vi "VelocityControl.vi"(0 "estimatives":T3, 1 "Dest_orientation":dbl, 2 "Position":dbl[](array[numeric]), 3 "Waypoint 1":dbl[](array[numeric]), 4 "Waypoint 0":dbl[](array[numeric]), 5 "Vx":dbl format="%#_13g", 7 "PID gains Vel":T2={"proportional gain (Kc)"=0.6, "integral time (Ti, min)"=0.0, "derivative time (Td, min)"=0.0}, 9 "Vy":dbl format="%#_13g", 11 "output xy":dbl=2.4, 12 "output inc":dbl=2.4, 13 "output angle":dbl=4.0, 14 "PID Gains Angle":T2={"proportional gain (Kc)"=5.0, "integral time (Ti, min)"=0.0, "derivative time (Td, min)"=-2.0}) -> (8 "Output Velocity":dbl[](array[numeric]) format="%.2f")   [LabVIEW 2018]
uses:
  Controle/VelocityGraph.ctl
  <vilib>/Analysis/coordinate.llb/Wrap Angle (scalar).vi
  <vilib>/Analysis/coordinate.llb/2D Cartesian Coordinate Rotation (Scalar).vi
  <vilib>/Analysis/NI_AAL_Angle.lvlib
  <vilib>/Analysis/NI_AALPro.lvlib
panel:
  out "Velocity Y":T1
  out "Velocity X":T1
  in  "Reinitialize":bool
  in  "PID Gains lateral":T2={"proportional gain (Kc)"=10.0, "integral time (Ti, min)"=0.0, "derivative time (Td, min)"=0.0}
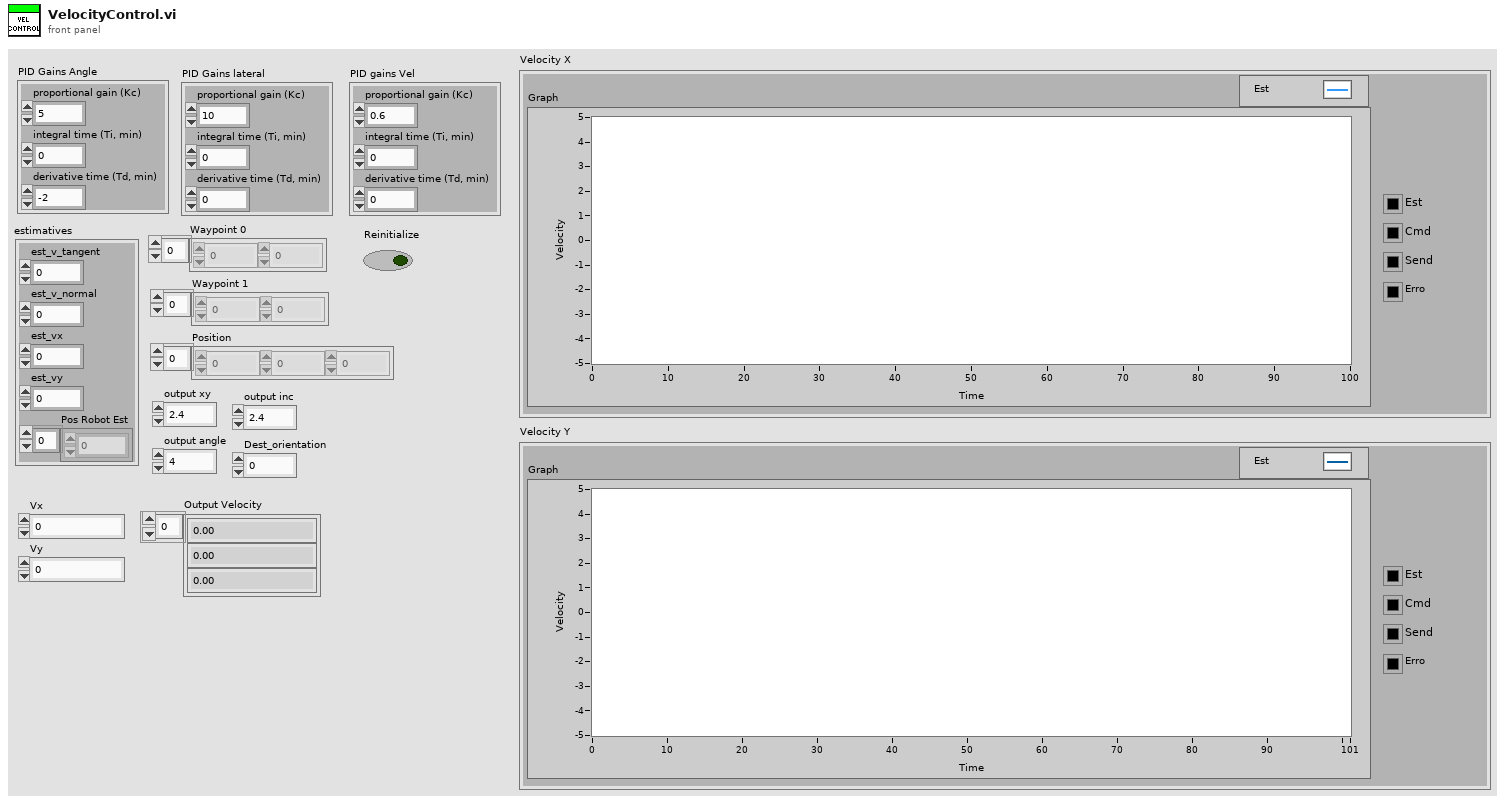
[diagram p1: front panel]
types:
  T1 = typedef "VelocityGraph.ctl" = cluster{"Graph":cluster{"est_vx":dbl, "Vx":dbl, dbl, "x out":dbl}, "Est":u32, "Cmd":u32, "Send":u32, "Erro":u32}
  T2 = cluster{"proportional gain (Kc)":dbl, "integral time (Ti, min)":dbl, "derivative time (Td, min)":dbl}
  T3 = cluster{"est_v_tangent":dbl, "est_v_normal":dbl, "est_vx":dbl, "est_vy":dbl, "Pos Robot Est":dbl[]}
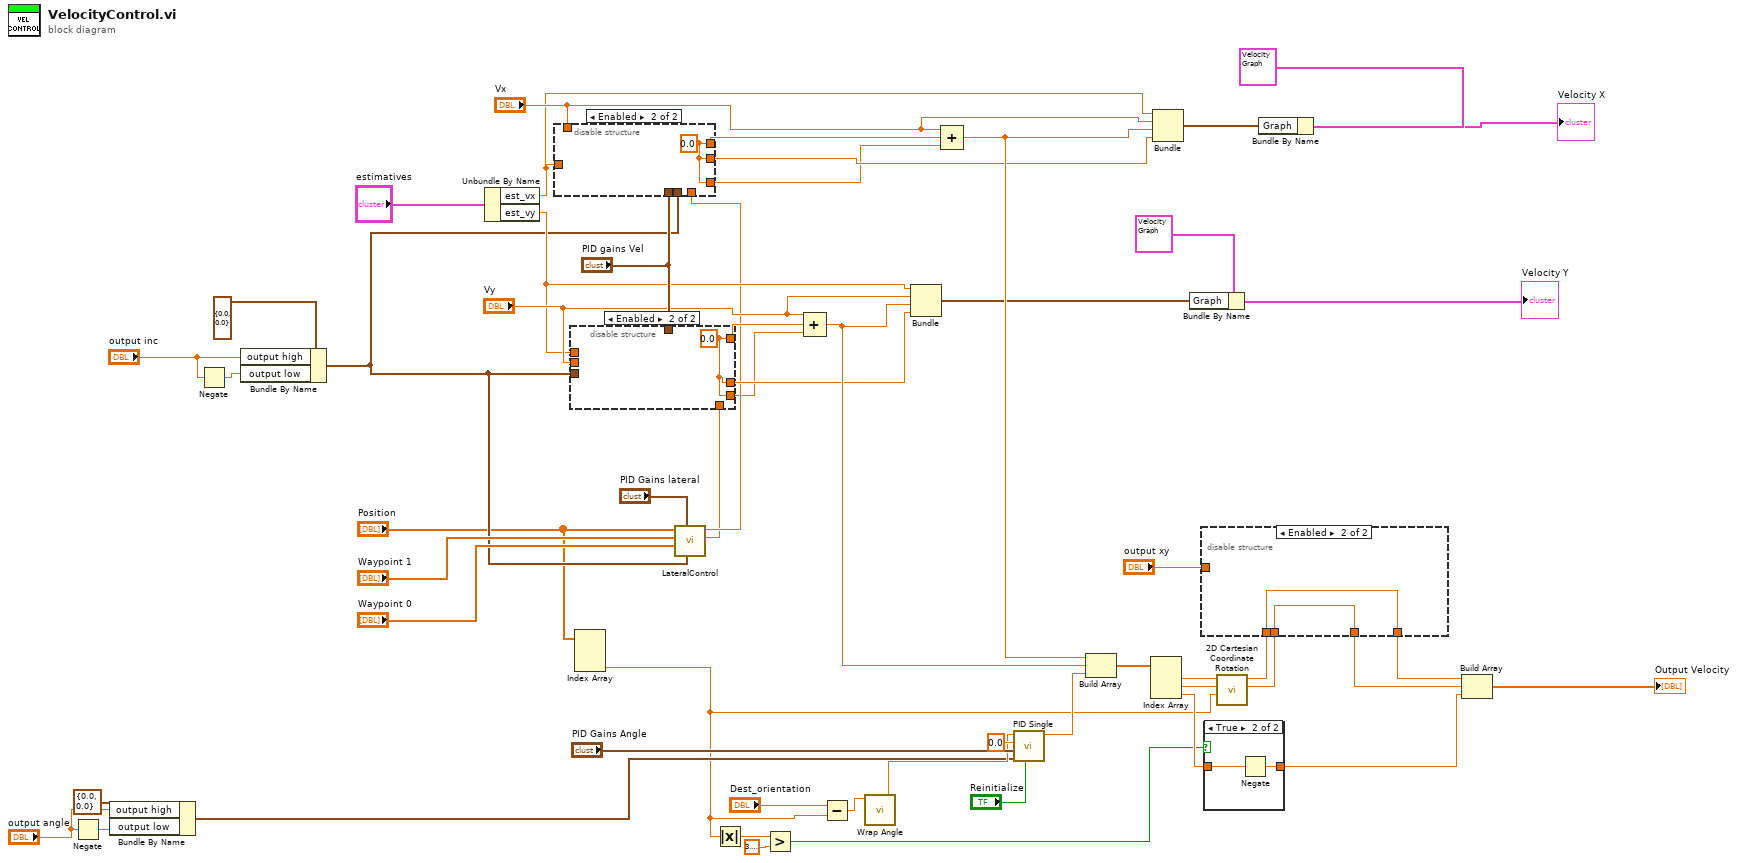
[diagram p0: block diagram]
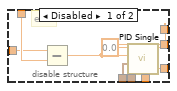
[diagram p2: hidden frame]
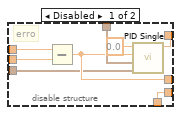
[diagram p3: hidden frame]
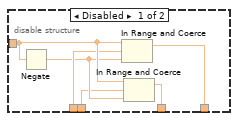
[diagram p4: hidden frame]
diagram:
  n1 = Negate(x="output angle") -> (-x=w42:dbl)
  n2 = Bundle By Name(cluster=cluster{"output high":dbl, "output low":dbl} {"output high"=0.0, "output low"=0.0}, "output high"="output angle", "output low"=w42) -> (w13:cluster{"output high":dbl, "output low":dbl})
  n3 = Negate(x="output inc") -> (-x=w25:dbl)
  n4 = Bundle By Name(cluster=cluster{"output high":dbl, "output low":dbl} {"output high"=0.0, "output low"=0.0} ("new element/subarray"), "output high"="output inc", "output low"=w25) -> (w12:cluster{"output high":dbl, "output low":dbl})
  n5 = Unbundle By Name("estimatives") -> ("est_vx"=w23:dbl, "est_vy"=w22:dbl)
  n6 = Index Array(array="Position") -> (element #3=w10:dbl)  [unwired: 3 in, 2 out]
  n7 = call "LateralControl.vi"("output range"=w12, "PID Gains lateral"="PID Gains lateral", "Waypoint 0"="Waypoint 0", "Waypoint 1"="Waypoint 1", "Position"="Position") -> ("y out"=w2:dbl, "x out"=w4:dbl)  [unwired: 5 in]
  n8 = disable-structure shown="Enabled" {
    disable-tunnel: [w63 w65] -> w33
    disable-tunnel: "PID gains Vel" -> [w62 _]
    disable-tunnel: "Vx" -> [w61 _]
    disable-tunnel: w23 -> [w60 _]
    disable-tunnel: [w59 w65] -> w15
    disable-tunnel: w12 -> [w58 _]
    disable-tunnel: w4 -> [w57 _]
    disable-tunnel: [w57 w65] -> w3
    frame Disabled {
      # "erro"
      n9 = Subtract(x=w60, y=w61) -> (x-y=w59:dbl)
      n10 = call "PID Single.vi"("Limits"=w58, "PID gains in"=w62, "Variable"=w59, "Setpoint"=0.0) -> ("Out"=w63:dbl)  [unwired: 7 in]
    }
    frame Enabled {
      w65 = 0.0 ("Out")
    }
  }
  n11 = disable-structure shown="Enabled" {
    disable-tunnel: [w73 w74] -> w32
    disable-tunnel: "PID gains Vel" -> [w71 _]
    disable-tunnel: "Vy" -> [w70 _]
    disable-tunnel: w22 -> [w69 _]
    disable-tunnel: [w68 w74] -> w14
    disable-tunnel: w12 -> [w67 _]
    disable-tunnel: w2 -> [w66 _]
    disable-tunnel: [w66 w74] -> w1
    frame Disabled {
      # "erro"
      n12 = Subtract(x=w69, y=w70) -> (x-y=w68:dbl)
      n13 = call "PID Single.vi"("Limits"=w67, "PID gains in"=w71, "Variable"=w68, "Setpoint"=0.0) -> ("Out"=w73:dbl)  [unwired: 7 in]
    }
    frame Enabled {
      w74 = 0.0 ("Out")
    }
  }
  n14 = Absolute Value(x=w10) -> (abs(x)=w54:dbl)
  n15 = Greater?(x=w54, y=3.141592653589793) -> (0:w49:bool)
  n16 = Compound Arithmetic op=ADD("Vy", w32, w1) -> (w27:dbl)
  n17 = Subtract(x="Dest_orientation", y=w10) -> (x-y=w46:dbl)
  n18 = call-poly <vilib>:"Wrap Angle.vi"("angle in"=w46) -> ("angle out"=w45:dbl)  [unwired: 9 in, 1 out]
  n19 = Bundle("est_vy"=w22, "Vy"="Vy", w27, "Out"=w14) -> (w20:cluster{"est_vy":dbl, "Vy":dbl, dbl, "Out":dbl})  [unwired: 1 in]
  n20 = Compound Arithmetic op=ADD("Vx", w33, w3) -> (w29:dbl)
  n21 = call "PID Single.vi"("initialize"="Reinitialize", "Limits"=w13, "PID gains in"="PID Gains Angle", "Variable"=0.0, "Setpoint"=w45) -> ("Out"=w50:dbl)  [unwired: 6 in]
  n22 = Build Array(w29, w27, w50) -> (w44:dbl[])
  n23 = Index Array(array=w44) -> (element #1=w56:dbl, element #2=w55:dbl, element #3=w53:dbl)  [unwired: 3 in]
  n24 = Bundle("est_vx"=w23, "Vx"="Vx", w29, "Out"=w15) -> (w17:cluster{"est_vx":dbl, "Vx":dbl, dbl, "Out":dbl})  [unwired: 1 in]
  n25 = Bundle By Name(cluster=T1 {"Graph"={"est_vx"=-0.14571416207204627, "Vx"=0.4692407651588243, 1.5797768746041183, "x out"=1.110536109445294}, "Est"=16860, "Cmd"=16711680, "Send"=6618880, "Erro"=16776722} ("Velocity Y"), "Graph"=w20) -> (→"Velocity Y":T1)
  n26 = case shown="True" w49 {
    tunnel: w53 -> [w75 w77]
    tunnel: [w75 w76] -> w52
    frame False {
    }
    frame True {
      n27 = Negate(x=w77) -> (-x=w76:dbl)
    }
  }
  n28 = call-poly <vilib>:"2D Cartesian Coordinate Rotation.vi"("theta"=w10, "y"=w55, "x"=w56) -> ("y out"=w7:dbl, "x out"=w8:dbl)  [unwired: 6 in, 1 out]
  n29 = disable-structure shown="Enabled" {
    disable-tunnel: "output xy" -> [w83 _]
    disable-tunnel: w8 -> [w82 w85]
    disable-tunnel: w7 -> [w80 w84]
    disable-tunnel: [w79 w85] -> w6
    disable-tunnel: [w78 w84] -> w5
    frame Disabled {
      n30 = Negate(x=w83) -> (-x=w81:dbl)
      n31 = In Range and Coerce(upper limit=w83, x=w82, lower limit=w81) -> (coerced(x)=w79:dbl)  [unwired: 1 out]
      n32 = In Range and Coerce(upper limit=w83, x=w80, lower limit=w81) -> (coerced(x)=w78:dbl)  [unwired: 1 out]
    }
    frame Enabled {
    }
  }
  n33 = Bundle By Name(cluster=T1 {"Graph"={"est_vx"=-0.14571416207204627, "Vx"=0.4692407651588243, 1.5797768746041183, "x out"=1.110536109445294}, "Est"=16860, "Cmd"=16711680, "Send"=6618880, "Erro"=16776722} ("Velocity Y"), "Graph"=w17) -> (→"Velocity X":T1)
  n34 = Build Array(w6, w5, w52) -> (→"Output Velocity":dbl[])
